vi "采配水公共部分.vi"() -> ()   [LabVIEW 2016, in "PLC.lvlib"]
uses:
  PLC.lvlib
panel:
  out "Registers":u16[](array[numeric])
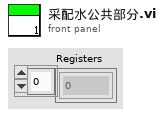
[diagram p1: front panel]
types:
  T1 = typedef "采配水类型.ctl" = enum16{"V1", "V2", "V3", "V4", "室内V1", "室内V2", "固定站V1", "固定站V2", "浮船V1", "浮船V2"}
  T2 = cluster{"R100":i16, "R101":i16, "R102":i16, "R103":i16, "R104":i16, "R105":i16, "R106":i16, "R107":i16, "R108":i16, "R109":i16, "R110":i16, "R111":i16, "R112":i16, "R113":i16, "R114":i16, "R115":i16, "R116":i16, "R117":i16, "R118":i16, "R119":i16, "R120":i16, "R121":i16, "R122":i16, "R123":i16, "R124":i16, "R125":i16, "R126":i16, "R127":i16, "R128":i16, "R129":i16, "R130":i16, "R131":i16, "R132":i16, "R133":i16}
  T3 = cluster{"配水时间":dbl, "沉淀时间":dbl, "清洗时间":dbl, "关键参数改变":bool}
  T4 = cluster{"状态":cluster{"R0":i16, "R1":i16, "R2":i16, "R3":i16, "R4":i16, "R5":i16, "R6":i16, "R7":i16, "R8":i16, "R9":i16, "R10":i16, "R11":i16, "R12":i16, "R13":i16, "R14":i16, "R15":i16, "R16":i16, "R17":i16, "R18":i16, "R19":i16, "R20":i16, "R21":i16, "R22":i16, "R23":i16, "R24":i16, "R25":i16, "R26":i16, "R27":i16, "R28":i16, "R29":i16, "R30":i16, "R31":i16, "R32":i16, "R33":i16, "R34":i16, "R35":i16, "R36":i16, "R37":i16, "R38":i16, "R39":i16}, "输入状态":bool[], "输出状态":bool[], "参数设置":cluster{"R100":i16, "R101":i16, "R102":i16, "R103":i16, "R104":i16, "R105":i16, "R106":i16, "R107":i16, "R108":i16, "R109":i16, "R110":i16, "R111":i16, "R112":i16, "R113":i16, "R114":i16, "R115":i16, "R116":i16, "R117":i16, "R118":i16, "R119":i16, "R120":i16, "R121":i16, "R122":i16, "R123":i16}, "转换值":cluster{"AD0":sgl, "AD1":sgl, "AD2":sgl, "AD3":sgl, "AD4":sgl, "AD5":sgl}}
  T5 = typedef "氨氮总磷总氮模块版本.ctl" = enum16{"V2", "V3"}
  T6 = cluster{"R0":i16, "R1":i16, "R2":i16, "R3":i16, "R4":i16, "R5":i16, "R6":i16, "R7":i16, "R8":i16, "R9":i16, "R10":i16, "R11":i16, "R12":i16, "R13":i16, "R14":i16, "R15":i16, "R16":i16, "R17":i16, "R18":i16, "R19":i16, "R20":i16, "R21":i16, "R22":i16, "R23":i16, "R24":i16, "R25":i16, "R26":i16, "R27":i16, "R28":i16, "R29":i16, "R30":i16, "R31":i16, "R32":i16, "R33":i16, "R34":i16, "R35":i16, "R36":i16, "R37":i16, "R38":i16, "R39":i16, "R40":i16, "R41":i16, "R42":i16, "R43":i16, "R44":i16, "R45":i16, "R46":i16, "R47":i16, "R48":i16, "R49":i16, "R50":i16, "R51":i16, "R52":i16, "R53":i16, "R54":i16, "R55":i16, "R56":i16, "R57":i16, "R58":i16, "R59":i16, "R60":i16, "R61":i16, "R62":i16, "R63":i16, "R64":i16, "R65":i16, "R66":i16, "R67":i16, "R68":i16, "R69":i16, "R70":i16, "R71":i16, "R72":i16, "R73":i16, "R74":i16, "R75":i16, "R76":i16, "R77":i16, "R78":i16, "R79":i16}
  T7 = cluster{"AD0":sgl, "AD1":sgl, "AD2":sgl, "AD3":sgl, "AD4":sgl, "AD5":sgl}
  T8 = cluster{"状态[0]":i16, "状态[1]":i16, "状态[2]":i16, "状态[3]":i16, "状态[4]":i16, "状态[5]":i16, "状态[6]":i16, "状态[7]":i16, "状态[8]":i16, "状态[9]":i16, "状态[10]":i16, "状态[11]":i16, "状态[12]":i16, "状态[13]":i16, "状态[14]":i16, "状态[15]":i16, "状态[16]":i16, "状态[17]":i16, "状态[18]":i16, "状态[19]":i16, "状态[20]":i16, "状态[21]":i16, "状态[22]":i16, "状态[23]":i16, "状态[24]":i16, "状态[25]":i16, "状态[26]":i16, "状态[27]":i16, "状态[28]":i16, "状态[29]":i16, "状态[30]":i16, "状态[31]":i16, "状态[32]":i16, "状态[33]":i16, "状态[34]":i16, "状态[35]":i16, "状态[36]":i16, "状态[37]":i16, "状态[38]":i16, "状态[39]":i16}
  T9 = cluster{"参数设置[0]":i16, "参数设置[1]":i16, "参数设置[2]":i16, "参数设置[3]":i16, "参数设置[4]":i16, "参数设置[5]":i16, "参数设置[6]":i16, "参数设置[7]":i16, "参数设置[8]":i16, "参数设置[9]":i16, "参数设置[10]":i16, "参数设置[11]":i16, "参数设置[12]":i16, "参数设置[13]":i16, "参数设置[14]":i16, "参数设置[15]":i16, "参数设置[16]":i16, "参数设置[17]":i16, "参数设置[18]":i16, "参数设置[19]":i16, "参数设置[20]":i16, "参数设置[21]":i16, "参数设置[22]":i16, "参数设置[23]":i16}
  T10 = cluster{"状态":cluster{"R0":i16, "R1":i16, "R2":i16, "R3":i16, "R4":i16, "R5":i16, "R6":i16, "R7":i16, "R8":i16, "R9":i16, "R10":i16, "R11":i16, "R12":i16, "R13":i16, "R14":i16, "R15":i16, "R16":i16, "R17":i16, "R18":i16, "R19":i16, "R20":i16, "R21":i16, "R22":i16, "R23":i16, "R24":i16, "R25":i16, "R26":i16, "R27":i16, "R28":i16, "R29":i16, "R30":i16, "R31":i16, "R32":i16, "R33":i16, "R34":i16, "R35":i16, "R36":i16, "R37":i16, "R38":i16, "R39":i16, "R40":i16, "R41":i16, "R42":i16, "R43":i16, "R44":i16, "R45":i16, "R46":i16, "R47":i16, "R48":i16, "R49":i16, "R50":i16, "R51":i16, "R52":i16, "R53":i16, "R54":i16, "R55":i16, "R56":i16, "R57":i16, "R58":i16, "R59":i16, "R60":i16, "R61":i16, "R62":i16, "R63":i16, "R64":i16, "R65":i16, "R66":i16, "R67":i16, "R68":i16, "R69":i16}, "输入状态":bool[], "输出状态":bool[], "报警簇":bool[], "参数设置":cluster{"R100":i16, "R101":i16, "R102":i16, "R103":i16, "R104":i16, "R105":i16, "R106":i16, "R107":i16, "R108":i16, "R109":i16, "R110":i16, "R111":i16, "R112":i16, "R113":i16, "R114":i16, "R115":i16, "R116":i16, "R117":i16, "R118":i16, "R119":i16, "R120":i16, "R121":i16, "R122":i16, "R123":i16, "R124":i16}, "转换值":cluster{"AD0":sgl, "AD1":sgl, "AD2":sgl, "AD3":sgl, "AD4":sgl, "AD5":sgl}, "看门狗启用":bool, "氨氮模块名称":string, "总磷模块名称":string, "采配水模块类型":enum16{"V1", "V2", "V3", "V4", "室内V1", "室内V2"}}
  T11 = cluster{"状态[0]":i16, "状态[1]":i16, "状态[2]":i16, "状态[3]":i16, "状态[4]":i16, "状态[5]":i16, "状态[6]":i16, "状态[7]":i16, "状态[8]":i16, "状态[9]":i16, "状态[10]":i16, "状态[11]":i16, "状态[12]":i16, "状态[13]":i16, "状态[14]":i16, "状态[15]":i16, "状态[16]":i16, "状态[17]":i16, "状态[18]":i16, "状态[19]":i16, "状态[20]":i16, "状态[21]":i16, "状态[22]":i16, "状态[23]":i16, "状态[24]":i16, "状态[25]":i16, "状态[26]":i16, "状态[27]":i16, "状态[28]":i16, "状态[29]":i16, "状态[30]":i16, "状态[31]":i16, "状态[32]":i16, "状态[33]":i16, "状态[34]":i16, "状态[35]":i16, "状态[36]":i16, "状态[37]":i16, "状态[38]":i16, "状态[39]":i16, "状态[40]":i16, "状态[41]":i16, "状态[42]":i16, "状态[43]":i16, "状态[44]":i16, "状态[45]":i16, "状态[46]":i16, "状态[47]":i16, "状态[48]":i16, "状态[49]":i16, "状态[50]":i16, "状态[51]":i16, "状态[52]":i16, "状态[53]":i16, "状态[54]":i16, "状态[55]":i16, "状态[56]":i16, "状态[57]":i16, "状态[58]":i16, "状态[59]":i16, "状态[60]":i16, "状态[61]":i16, "状态[62]":i16, "状态[63]":i16, "状态[64]":i16, "状态[65]":i16, "状态[66]":i16, "状态[67]":i16, "状态[68]":i16, "状态[69]":i16}
  T12 = cluster{"参数设置[0]":i16, "参数设置[1]":i16, "参数设置[2]":i16, "参数设置[3]":i16, "参数设置[4]":i16, "参数设置[5]":i16, "参数设置[6]":i16, "参数设置[7]":i16, "参数设置[8]":i16, "参数设置[9]":i16, "参数设置[10]":i16, "参数设置[11]":i16, "参数设置[12]":i16, "参数设置[13]":i16, "参数设置[14]":i16, "参数设置[15]":i16, "参数设置[16]":i16, "参数设置[17]":i16, "参数设置[18]":i16, "参数设置[19]":i16, "参数设置[20]":i16, "参数设置[21]":i16, "参数设置[22]":i16, "参数设置[23]":i16, "参数设置[24]":i16}
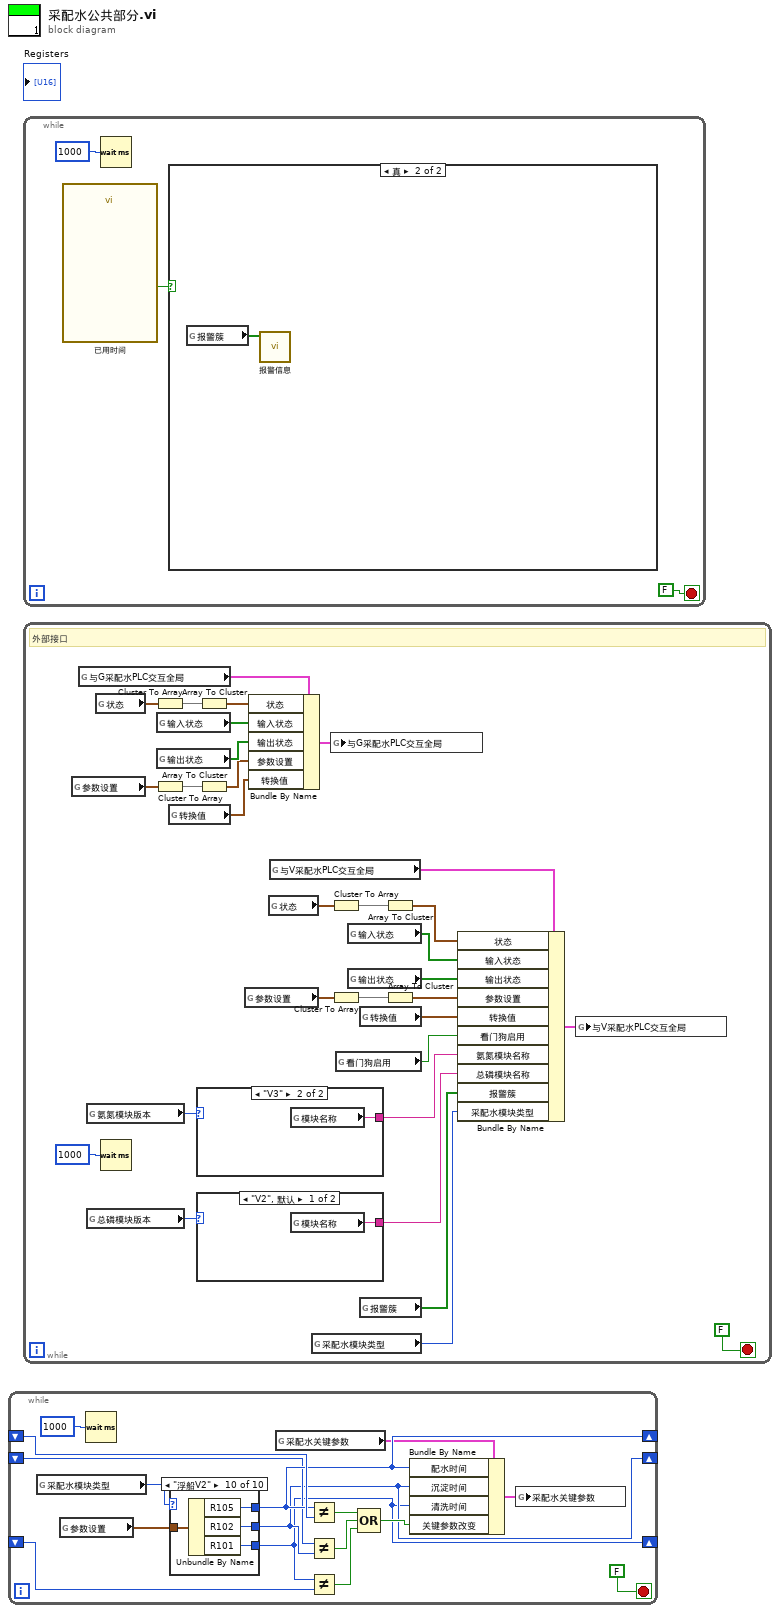
[diagram p0: block diagram]
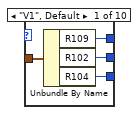
[diagram p2: hidden frame]
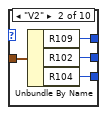
[diagram p3: hidden frame]
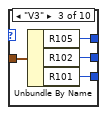
[diagram p4: hidden frame]
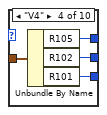
[diagram p5: hidden frame]
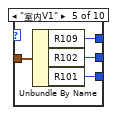
[diagram p6: hidden frame]
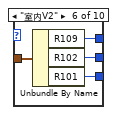
[diagram p7: hidden frame]
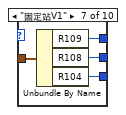
[diagram p8: hidden frame]
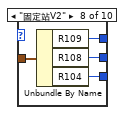
[diagram p9: hidden frame]
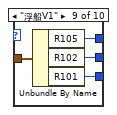
[diagram p10: hidden frame]
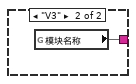
[diagram p12: hidden frame]
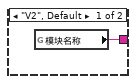
[diagram p13: hidden frame]
diagram:
  n1 = while {
    shift-right: [w13] -> _
    shift-left: _ -> [w14]
    shift-right: [w4] -> _
    shift-left: _ -> [w10]
    shift-right: [w3] -> _
    shift-left: _ -> [w8]
    stop <- FALSE stop-if-true
    n2 = global read "系统设置全局变量.vi" "采配水模块类型"() -> (w16:T1)
    n3 = global read "采配水全局变量.vi" "参数设置"() -> (w15:T2)
    n4 = Wait (ms)(milliseconds to wait=u32 1000 ("等待时间（毫秒）")) -> ()  [unwired: 1 out]
    n5 = case shown="\"浮船V2\"" w16 {
      tunnel: w15 -> [w20 w24 w27 w32 w36 w40 w44 w48 w52 w56]
      tunnel: [w19 w23 w28 w31 w35 w39 w43 w47 w51 w55] -> w13
      tunnel: [w18 w22 w25 w30 w34 w38 w42 w46 w50 w54] -> w4
      tunnel: [w17 w21 w26 w29 w33 w37 w41 w45 w49 w53] -> w3
      frame "V1", Default {
        n6 = Unbundle By Name(w20) -> ("R109"=w19:i16, "R102"=w18:i16, "R104"=w17:i16)
      }
      frame "V2" {
        n7 = Unbundle By Name(w24) -> ("R109"=w23:i16, "R102"=w22:i16, "R104"=w21:i16)
      }
      frame "V3" {
        n8 = Unbundle By Name(w27) -> ("R105"=w28:i16, "R102"=w25:i16, "R101"=w26:i16)
      }
      frame "V4" {
        n9 = Unbundle By Name(w32) -> ("R105"=w31:i16, "R102"=w30:i16, "R101"=w29:i16)
      }
      frame "室内V1" {
        n10 = Unbundle By Name(w36) -> ("R109"=w35:i16, "R102"=w34:i16, "R101"=w33:i16)
      }
      frame "室内V2" {
        n11 = Unbundle By Name(w40) -> ("R109"=w39:i16, "R102"=w38:i16, "R101"=w37:i16)
      }
      frame "固定站V1" {
        n12 = Unbundle By Name(w44) -> ("R109"=w43:i16, "R108"=w42:i16, "R104"=w41:i16)
      }
      frame "固定站V2" {
        n13 = Unbundle By Name(w48) -> ("R109"=w47:i16, "R108"=w46:i16, "R104"=w45:i16)
      }
      frame "浮船V1" {
        n14 = Unbundle By Name(w52) -> ("R105"=w51:i16, "R102"=w50:i16, "R101"=w49:i16)
      }
      frame "浮船V2" {
        n15 = Unbundle By Name(w56) -> ("R105"=w55:i16, "R102"=w54:i16, "R101"=w53:i16)
      }
    }
    n16 = global read "采配水全局变量.vi" "采配水关键参数"() -> (w1:T3)
    n17 = Not Equal?(x=w13, y=w14) -> (x != y?=w11:bool)
    n18 = Not Equal?(x=w10, y=w4) -> (x != y?=w9:bool)
    n19 = Not Equal?(x=w3, y=w8) -> (x != y?=w7:bool)
    n20 = Compound Arithmetic op=OR ("复合运算")(w11, w9, w7) -> (w12:bool)
    n21 = Bundle By Name(cluster=w1, "配水时间"=w13, "沉淀时间"=w4, "清洗时间"=w3, "关键参数改变"=w12) -> (w2:T3)
    n22 = global write "采配水全局变量.vi" "采配水关键参数"(w2) -> ()
  }
  n23 = while {
    stop <- FALSE stop-if-true
    n24 = call "已用时间"() -> ("Time has Elapsed"=w59:bool)  [unwired: 12 in, 7 out]
    n25 = Wait (ms)(milliseconds to wait=u32 1000 ("等待时间（毫秒）")) -> ()  [unwired: 1 out]
    n26 = case shown="真" w59 {
      frame False {
      }
      frame True {
        n27 = global read "采配水全局变量.vi" "报警簇"() -> (w60:bool[])
        n28 = call "报警信息.vi"("报警簇"=w60) -> ()  [unwired: 9 in, 2 out]
      }
    }
  }
  n29 = while {
    stop <- FALSE stop-if-true
    # "外部接口"
    n30 = global read "采配水全局变量.vi" "参数设置"() -> (w68:T2)
    n31 = global read "外部交互全局变量.vi" "与G采配水PLC交互全局"() -> (w75:T4)
    n32 = global read "系统设置全局变量.vi" "氨氮模块版本"() -> (w64:T5)
    n33 = global read "系统设置全局变量.vi" "总磷模块版本"() -> (w63:T5)
    n34 = global read "采配水全局变量.vi" "状态"() -> (w72:T6)
    n35 = Wait (ms)(milliseconds to wait=u32 1000 ("等待时间（毫秒）")) -> ()  [unwired: 1 out]
    n36 = Cluster To Array(cluster=w72) -> (array=w73:i16[])
    n37 = Cluster To Array(cluster=w68) -> (array=w67:i16[])
    n38 = global read "采配水全局变量.vi" "输入状态"() -> (w70:bool[])
    n39 = global read "采配水全局变量.vi" "输出状态"() -> (w69:bool[])
    n40 = global read "采配水全局变量.vi" "转换值"() -> (w66:T7)
    n41 = case shown="\"V3\"" w64 {
      tunnel: [w94 w95] -> w62
      frame "V2", Default {
        n42 = global read "VAR总磷总氮全局变量.vi" "模块名称"() -> (w94:string)
      }
      frame "V3" {
        n43 = global read "VAR总磷总氮全局变量.vi" "模块名称"() -> (w95:string)
      }
    }
    n44 = case shown="\"V2\", 默认" w63 {
      tunnel: [w92 w93] -> w61
      frame "V2", Default {
        n45 = global read "VAR总磷总氮全局变量.vi" "模块名称"() -> (w92:string)
      }
      frame "V3" {
        n46 = global read "VAR总磷总氮全局变量.vi" "模块名称"() -> (w93:string)
      }
    }
    n47 = Array To Cluster(array=w73) -> (cluster=w71:T8)
    n48 = Array To Cluster(array=w67) -> (cluster=w65:T9)
    n49 = global read "采配水全局变量.vi" "参数设置"() -> (w78:T2)
    n50 = Bundle By Name(cluster=w75, "状态"=w71, "输入状态"=w70, "输出状态"=w69, "参数设置"=w65, "转换值"=w66) -> (w74:T4)
    n51 = global read "采配水全局变量.vi" "状态"() -> (w82:T6)
    n52 = global read "外部交互全局变量.vi" "与V采配水PLC交互全局"() -> (w89:T10)
    n53 = global read "系统设置全局变量.vi" "采配水模块类型"() -> (w76:T1)
    n54 = global write "外部交互全局变量.vi" "与G采配水PLC交互全局"(w74) -> ()
    n55 = Cluster To Array(cluster=w82) -> (array=w81:i16[])
    n56 = Cluster To Array(cluster=w78) -> (array=w79:i16[])
    n57 = global read "采配水全局变量.vi" "看门狗启用"() -> (w84:bool)
    n58 = global read "采配水全局变量.vi" "输入状态"() -> (w88:bool[])
    n59 = global read "采配水全局变量.vi" "输出状态"() -> (w87:bool[])
    n60 = global read "采配水全局变量.vi" "转换值"() -> (w86:T7)
    n61 = global read "采配水全局变量.vi" "报警簇"() -> (w83:bool[])
    n62 = Array To Cluster(array=w81) -> (cluster=w80:T11)
    n63 = Array To Cluster(array=w79) -> (cluster=w77:T12)
    n64 = Bundle By Name(cluster=w89, "状态"=w80, "输入状态"=w88, "输出状态"=w87, "参数设置"=w77, "转换值"=w86, "看门狗启用"=w84, "氨氮模块名称"=w62, "总磷模块名称"=w61, "报警簇"=w83, "采配水模块类型"=w76) -> (w85:T10)
    n65 = global write "外部交互全局变量.vi" "与V采配水PLC交互全局"(w85) -> ()
  }
